vi "PutFixStr.vi"(8 "error in (no error)":errorcluster, 9 "Size":i32, 10 "string":string, 11 "MsgPackSerializer in":refnum<class "MsgPackSerializer.lvclass">) -> (0 "error out":errorcluster, 3 "MsgPackSerializer out":refnum<class "MsgPackSerializer.lvclass">)   [LabVIEW 2015, in "MsgPackSerializer.lvclass"]
uses:
  MsgPackSerializer.lvclass
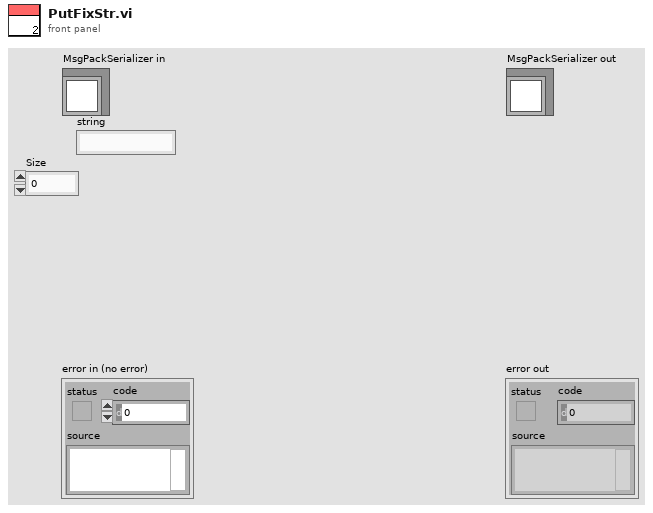
[diagram p1: front panel]
types:
  T1 = enum16{"big-endian, network order", "native, host order", "little-endian"}
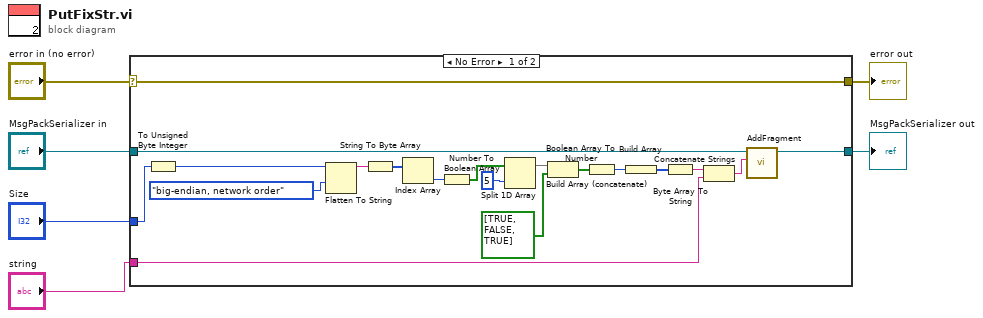
[diagram p0: block diagram]
diagram:
  n1 = case shown="No Error" "error in (no error)" {
    selector: "error in (no error)" -> [w25 w27]
    tunnel: [w25 w27] -> w5
    tunnel: [w23 w26] -> w3
    tunnel: "MsgPackSerializer in" -> [w24 w26]
    tunnel: "string" -> [w7 _]
    tunnel: "Size" -> [w9 _]
    frame No Error {
      n2 = To Unsigned Byte Integer(number=w9) -> (unsigned 8bit integer=w18:u8)
      n3 = Flatten To String(anything=w18, byte order (0:big-endian, network order)=T1."big-endian, network order") -> (data string=w17:string)  [unwired: 2 in, 2 out]
      n4 = String To Byte Array(string=w17) -> (unsigned byte array=w16:u8[])
      n5 = Index Array(array=w16) -> (element=w15:u8)  [unwired: 1 in]
      n6 = Number To Boolean Array(number=w15) -> (Boolean array=w22:bool[])
      n7 = Split 1D Array(array=w22, index=5) -> (first subarray=w20:bool[])  [unwired: 1 out]
      n8 = Build Array (concatenate)(w20, bool[] [TRUE, FALSE, TRUE] ("Boolean array")) -> (w13:bool[])
      n9 = Boolean Array To Number(Boolean array=w13) -> (number=w12:u32)
      n10 = Build Array(w12) -> (w11:u32[])
      n11 = Byte Array To String(unsigned byte array=w11) -> (string=w8:string)
      n12 = Concatenate Strings(w8, w7) -> (w10:string)
      n13 = call "AddFragment.vi"("Fragment"=w10, "MsgPackSerializer in"=w24) -> ("MsgPackSerializer out"=w23:refnum<class "MsgPackSerializer.lvclass">)  [unwired: 8 in, 1 out]
    }
    frame Error {
    }
  }
  "error out" <- w5
  "MsgPackSerializer out" <- w3
